vi "mod_PSK Transmitter.vi"(0 "Symbol Rate, Hz":dbl=1.0 format="%.2f", 1 "Reset?":bool=TRUE, 2 "# Samples per Symbol":i32=16, 5 "PSK":T1={"M-PSK (4)"=4, "differential PSK"=enum."disable", "PSK type"=0} {"PSK type" items=["normal", "shifted", "offset"]}, 7 "Message":T3={"# Guard Bits"=2, "# Sync Bits"=20, "# Message Bits"=1000, "PN sequence order"=9}, 9 "System Filter":T2={"TX Filter"=enum."Root Raised Cos", "Alpha"=0.5, "filter length"=8} {"Alpha" format="%.2f"}, 11 "error in (no error)":errorcluster) -> (4 "Output Complex Waveform":cluster{"t0":dbl, "dt":dbl, "Y":cdb[]} {"Y" format="%.3f"; "dt" format="%^.2e"; "t0" format="%.4f"}, 6 "Signal Description":T5 {"PSK system parameters"."PSK type" items=["normal", "shifted", "offset"]; "PSK system parameters"."symbol map" format="%.3f"; "matched filter coefficients" format="%.2f"; "pulse shaping filter coefficients" format="%.2f"; "Sync (Symbols)" format="%.2f"}, 15 "error out":errorcluster)   [LabVIEW 2020, in "niDMT.lvlib"]
doc: "This example demonstrates generation of a PSK modulated signal. You can specify characteristics of the message signal such as PN sequence order, number of guard bits, number of sync bits, and transmit filter parameters. You can extend this example to download the generated PSK signal to GPIB-based RF signal generators."
uses:
  <vilib>/addons/Modulation/niDMT.lvlib
  <vilib>/addons/Modulation/Digital/Support/Controls/PSK System Parameters.ctl
  <vilib>/addons/Modulation/Analog/support/mod_Set Error Source.vi
  <vilib>/addons/Modulation/Digital/Support/Common/Validators/mod_Generate Filter Coefficients Validate.vi
  <vilib>/addons/Modulation/Digital/General/subVIs/mod_Generate Filter Coefficients.vi
  <vilib>/addons/Modulation/Digital/General/MT Generate PSK System Parameters(M).vi
  <vilib>/addons/Modulation/Digital/General/MT Generate PSK Synchronization Parameters (bit array).vi
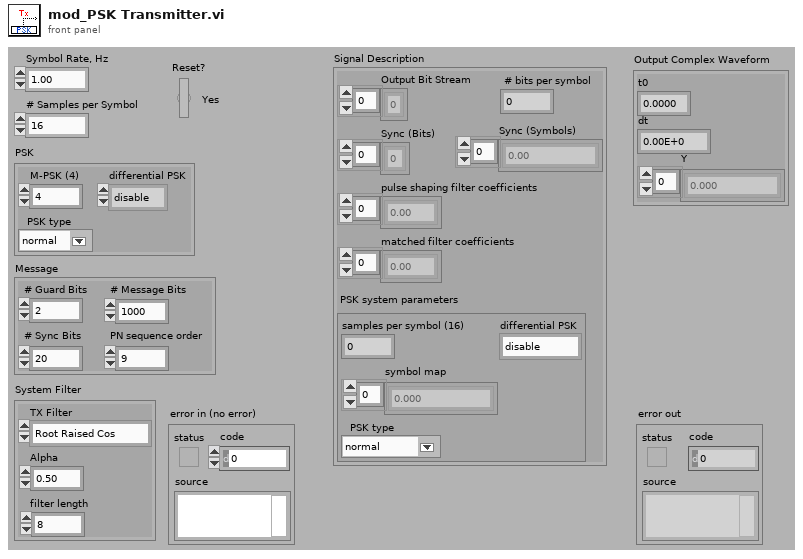
[diagram p1: front panel]
types:
  T1 = cluster{"M-PSK (4)":i32, "differential PSK":enum16{"disable", "enable"}, "PSK type":u16}
  T2 = cluster{"TX Filter":enum16{"none", "Raised Cosine", "Root Raised Cos", "Gaussian"}, "Alpha":dbl, "filter length":i32}
  T3 = cluster{"# Guard Bits":i32, "# Sync Bits":i32, "# Message Bits":i32, "PN sequence order":i32}
  T4 = typedef "niDMT.lvlib/PSK System Parameters.ctl" = cluster{"samples per symbol (16)":i32, "symbol map":cdb[], "differential PSK":enum16{"disable", "enable"}, "PSK type":u16}
  T5 = cluster{"Output Bit Stream":i8[], " # bits per symbol":i32, "Sync (Bits)":i8[], "Sync (Symbols)":cdb[], "pulse shaping filter coefficients":dbl[], "matched filter coefficients":dbl[], "PSK system parameters":T4}
  T6 = cluster{"Output Bit Stream":i8[], "# bits per symbol":i32, "Sync (Bits)":i8[], "Sync (Symbols)":cdb[], "pulse shaping filter coefficients":dbl[], "matched filter coefficients":dbl[], "PSK system parameters":T4}
  T7 = enum16{"none", "Raised Cosine", "Root Raised Cos", "Gaussian"}
  T8 = cluster{"samples per symbol (16)":i32, "symbol map":cdb[], "differential PSK":enum16{"disable", "enable"}, "PSK type":u16}
  T9 = cluster{"expected sync location (symbols)":i32, "sync sequence":cdb[], "sync location uncertainty (symbols)":i32, "sync indent (symbols)":i32}
  T10 = typedef "niAMT.lvlib/Complex Data Waveform.ctl" = cluster{"t0":dbl, "dt":dbl, "Y":cdb[]}
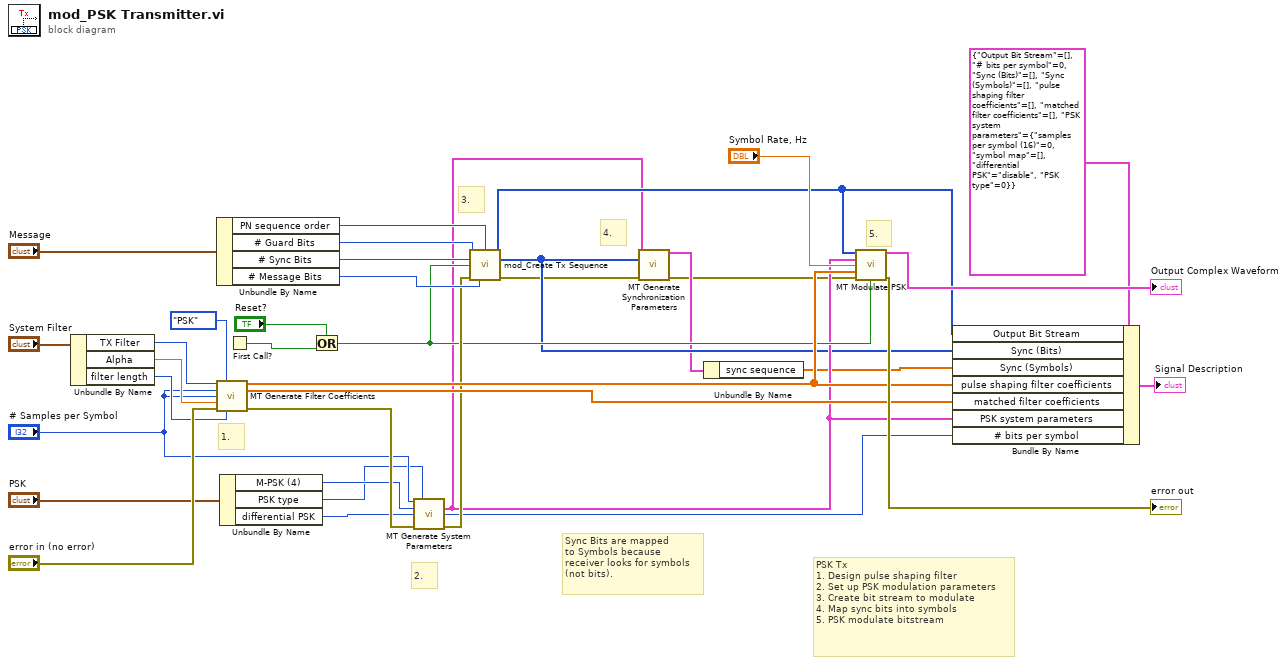
[diagram p0: block diagram]
diagram:
  # "5."
  # "4."
  # "2."
  # "3."
  # "1."
  # "PSK Tx\n1. Design pulse shaping filter\n2. Set up PSK modulation parameters\n3. Create bit stream to modulate\n4. Map sync bits into symbols\n5. PSK modulate bitstream"
  # "Sync Bits are mapped\nto Symbols because\nreceiver looks for symbols\n(not bits)."
  n1 = Unbundle By Name("System Filter") -> ("TX Filter"=w24:T7, "Alpha"=w23:dbl, "filter length"=w22:i32)
  n2 = Unbundle By Name("Message") -> ("PN sequence order"=w18:i32, "# Guard Bits"=w28:i32, "# Sync Bits"=w27:i32, "# Message Bits"=w26:i32)
  n3 = call <vilib>:"MT Generate Filter Coefficients.vi"("pulse shaping filter (none)"=w24, "modulation type"=enum16{"FSK", "PSK", "QAM", "MSK"}."PSK" ("Modulation Type"), "pulse shaping samples per symbol (16)"="# Samples per Symbol", "matched samples per symbol (16)"="# Samples per Symbol", "filter parameter"=w23, "error in (no error)"="error in (no error)", "filter length (symbols)"=w22) -> ("pulse shaping filter coefficients"=w20:dbl[], "matched filter coefficients"=w19:dbl[], "error out"=w14:errorcluster)  [unwired: 6 out]
  n4 = Unbundle By Name("PSK") -> ("M-PSK (4)"=w11:i32, "PSK type"=w9:u16, "differential PSK"=w7:enum16{"disable", "enable"})
  n5 = First Call?() -> (First Call?: T/F=w31:bool)
  n6 = Or(x="Reset?", y=w31) -> (x .or. y?=w8:bool)
  n7 = call-poly <vilib>:"MT Generate System Parameters.vi"("samples per symbol (16)"="# Samples per Symbol", "PSK type"=w9, "M-PSK (4)"=w11, "differential PSK"=w7, "error in (no error)"=w14) -> ("PSK system parameters"=w6:T8, "bits per symbol"=w12:i32, "error out"=w13:errorcluster)  [unwired: 8 out]
  n8 = call <vilib>:"mod_Create Tx Sequence.vi"("# Guard Bits (2)"=w28, "PN sequence order (9)"=w18, "# Sync Bits (20)"=w27, "Reset? (T)"=w8, "error in (no error)"=w13, "# Message Bits"=w26) -> ("Output Bit Stream"=w21:i8[], "Last Sync Pattern"=w5:i8[], "error out"=w3:errorcluster)  [unwired: 3 in, 4 out]
  n9 = call-poly <vilib>:"MT Generate Synchronization Parameters.vi"("PSK system parameters"=w6, "sync bits"=w5, "error in (no error)"=w3) -> ("PSK synchronization parameters"=w4:T9, "error out"=w1:errorcluster)  [unwired: 3 in, 8 out]
  n10 = Unbundle By Name(w4) -> ("sync sequence"=w2:cdb[])
  n11 = call <vilib>:"MT Modulate PSK.vi"("input bit stream"=w21, "PSK system parameters"=w6, "symbol rate (Hz)"="Symbol Rate, Hz", "pulse shaping filter coefficients"=w20, "error in (no error)"=w1, "reset? (T)"=w8) -> ("output complex waveform"=→"Output Complex Waveform":T10, "error out"=→"error out":errorcluster)  [unwired: 1 in, 7 out]
  n12 = Bundle By Name(cluster=T6 {"Output Bit Stream"=[], "# bits per symbol"=0, "Sync (Bits)"=[], "Sync (Symbols)"=[], "pulse shaping filter coefficients"=[], "matched filter coefficients"=[], "PSK system parameters"={"samples per symbol (16)"=0, "symbol map"=[], "differential PSK"=enum."disable", "PSK type"=0}} ("Signal Description"), "Output Bit Stream"=w21, "Sync (Bits)"=w5, "Sync (Symbols)"=w2, "pulse shaping filter coefficients"=w20, "matched filter coefficients"=w19, "PSK system parameters"=w6, "# bits per symbol"=w12) -> (→"Signal Description":T6)
